vi "write data chunk.vi"(8 "error in (no error)":errorcluster, 9 "pos offset (bytes:0)":i32, 10 "1D-array (chunk)":dbl[](array[numeric]) min=0.0 max=127.0 format="%.2f", 11 "Ref Num":refnum<file>) -> (0 "error out":errorcluster, 1 "mark after write (bytes)":i32, 3 "Dup Ref Num":refnum<file>)   [LabVIEW 2015]
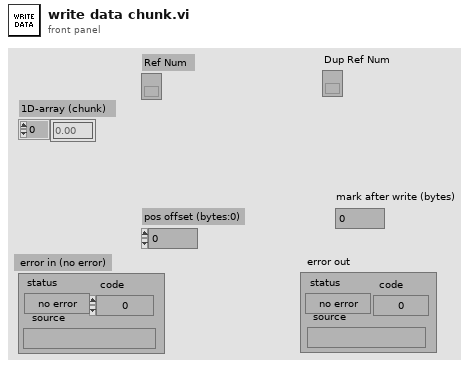
[diagram p1: front panel]
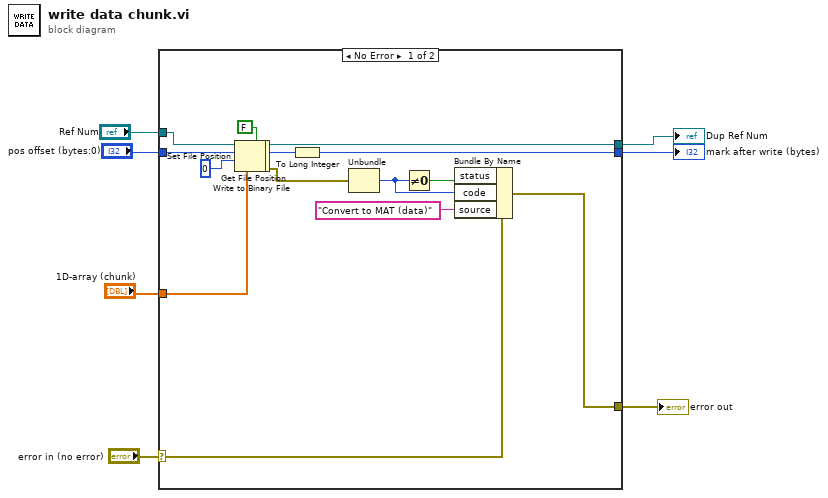
[diagram p0: block diagram]
diagram:
  n1 = case shown="No Error" "error in (no error)" {
    selector: "error in (no error)" -> [w8 w26]
    tunnel: [w23 w26] -> w7
    tunnel: [w22 w28] -> w5
    tunnel: "Ref Num" -> [w16 w28]
    tunnel: [w21 -1] -> w4
    tunnel: "1D-array (chunk)" -> [w18 _]
    tunnel: "pos offset (bytes:0)" -> [w17 _]
    frame No Error {
      n2 = Set File Position(offset (in bytes) (0)=w17, refnum=w16, from (0:start)=i16 0) -> (refnum out=w14:refnum<file>, error out=w13:errorcluster)  [unwired: 1 in]
      n3 = Write to Binary File(file (use dialog)=w14, data=w18, error in=w13, 5:FALSE ("prepend array or string size? (T)")) -> (refnum out=w12:refnum<file>, error out=w11:errorcluster)  [unwired: 2 in, 1 out]
      n4 = Get File Position(4:w11, 7:w12) -> (0:w19:errorcluster, 2:w10:i64, 3:w22:refnum<file>)
      n5 = To Long Integer(number=w10) -> (32bit integer=w21:i32)
      n6 = Unbundle(w19) -> ("code"=w20:i32)  [unwired: 2 out]
      n7 = Not Equal To 0?(x=w20) -> (x != 0?=w24:bool)
      n8 = Bundle By Name(cluster=w8, "status"=w24, "code"=w20, "source"="Convert to MAT (data)") -> (w23:errorcluster)
    }
    frame Error {
    }
  }
  "Dup Ref Num" <- w5
  "error out" <- w7
  "mark after write (bytes)" <- w4
